vi "ProgressBar.vi"(8 "msgIn":string="Creatng Grid", 9 "Progress":refnum<vi>) -> (1 "This VI":refnum<vi>)   [LabVIEW 2016]
panel:
  out "msgOut":string="Creating Grid"
  out "Creating grid":dbl(slide) scale=0.0..1.0
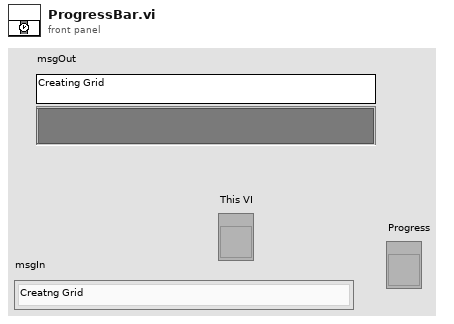
[diagram p1: front panel]
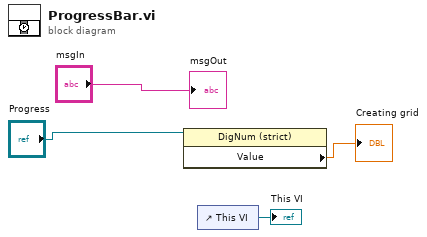
[diagram p0: block diagram]
diagram:
  n1 = property class="DigNum (strict)"(reference="Progress") -> ("Value"=→"Creating grid":dbl)  [unwired: 1 in, 2 out]
  n2 = control-ref of="This VI"() -> (→"This VI":refnum<vi>)
  "msgOut" <- "msgIn"
